vi "EDAFiltr(subVI).vi"(1 "Vstup":dbl format="%0.2f") -> (0 "Filtrovaný vstup":dbl format="%0.2f")   [LabVIEW 2026]
uses:
  <vilib>/ptbypt/NI_PtbyPt.lvlib
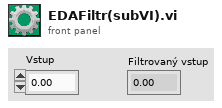
[diagram p1: front panel]
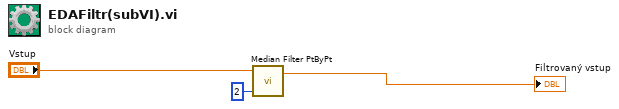
[diagram p0: block diagram]
diagram:
  n1 = call <vilib>:"Median Filter PtByPt.vi"("rank"=2, "x"="Vstup") -> ("Filtered x"=→"Filtrovaný vstup":dbl)  [unwired: 2 in, 1 out]
